vi "Generate New Word.vi"(10 "Exclude Previously Selected Words":bool, 11 "Used Words in":set{string}(c389)) -> (2 "Random Element":string, 3 "Used Words out":set{string}(c389))   [LabVIEW 2020, in "Wordle Engine.lvlib"]
uses:
  Wordle Engine.lvlib
  d95a550e-f149-4a10-be9d-5c03d5ffe434.vi
  <vilib>/numeric/sub_Random U32.vi
  <vilib>/numeric/Random Number (Range) U64.vi
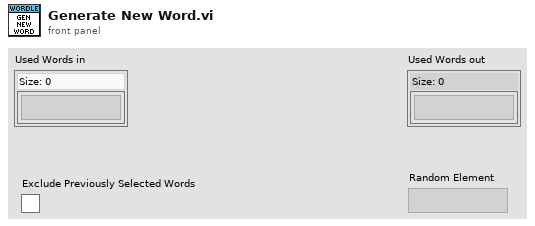
[diagram p1: front panel]
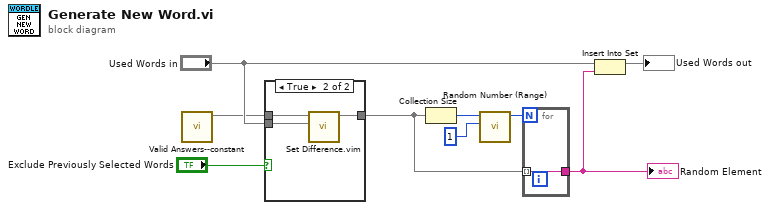
[diagram p0: block diagram]
diagram:
  n1 = call "Valid Answers--constant.vi"() -> ("Valid Answers"=w7:set{string})  [unwired: 11 in]
  n2 = case shown="True" "Exclude Previously Selected Words" {
    tunnel: "Used Words in" -> [_ w13]
    tunnel: w7 -> [w10 w12]
    tunnel: [w10 w11] -> w3
    frame False {
    }
    frame True {
      n3 = call "Set Difference.vim"("set 2"=w13, "set 1"=w12) -> ("difference"=w11:set{string})  [unwired: 9 in]
    }
  }
  n4 = Collection Size(1:w3) -> (0:w5:i32)
  n5 = call-poly <vilib>:"Random Number (Range).vi"("lower bound (0)"=u64 1, "upper bound (100)"=w5) -> ("number"=w4:u64)  [unwired: 9 in]
  n6 = for {
    N: w4 -> [_]
    tunnel: w3 -> [w14] mode=indexing
    tunnel: [w14] -> w2
  }
  "Random Element" <- w2
  n7 = Insert Into Set(10:w2, 11:"Used Words in") -> (3:→"Used Words out":set{string})  [unwired: 1 out]
